vi "Examen01.vi"() -> ()   [LabVIEW 2020]
uses:
  <vilib>/Instr/_visa.llb/VISA Configure Serial Port (Instr).vi
panel:
  out "Waveform Chart":dynamicdata(graph)
  out "Valor Mínimo (°C)":dbl
  out "Valor Máximo (°C)":dbl
  out "Dato actual (°C)":dbl
  in  "stop":bool
  in  "VISA resource name":refnum<visa-resource-name>
  # "SENSOR LM35"
  # "Señal original"
  # "Señal filtrada"
  # "Juan Daniel Magdaleno Arellano\nLuis David Casas Hernandez"
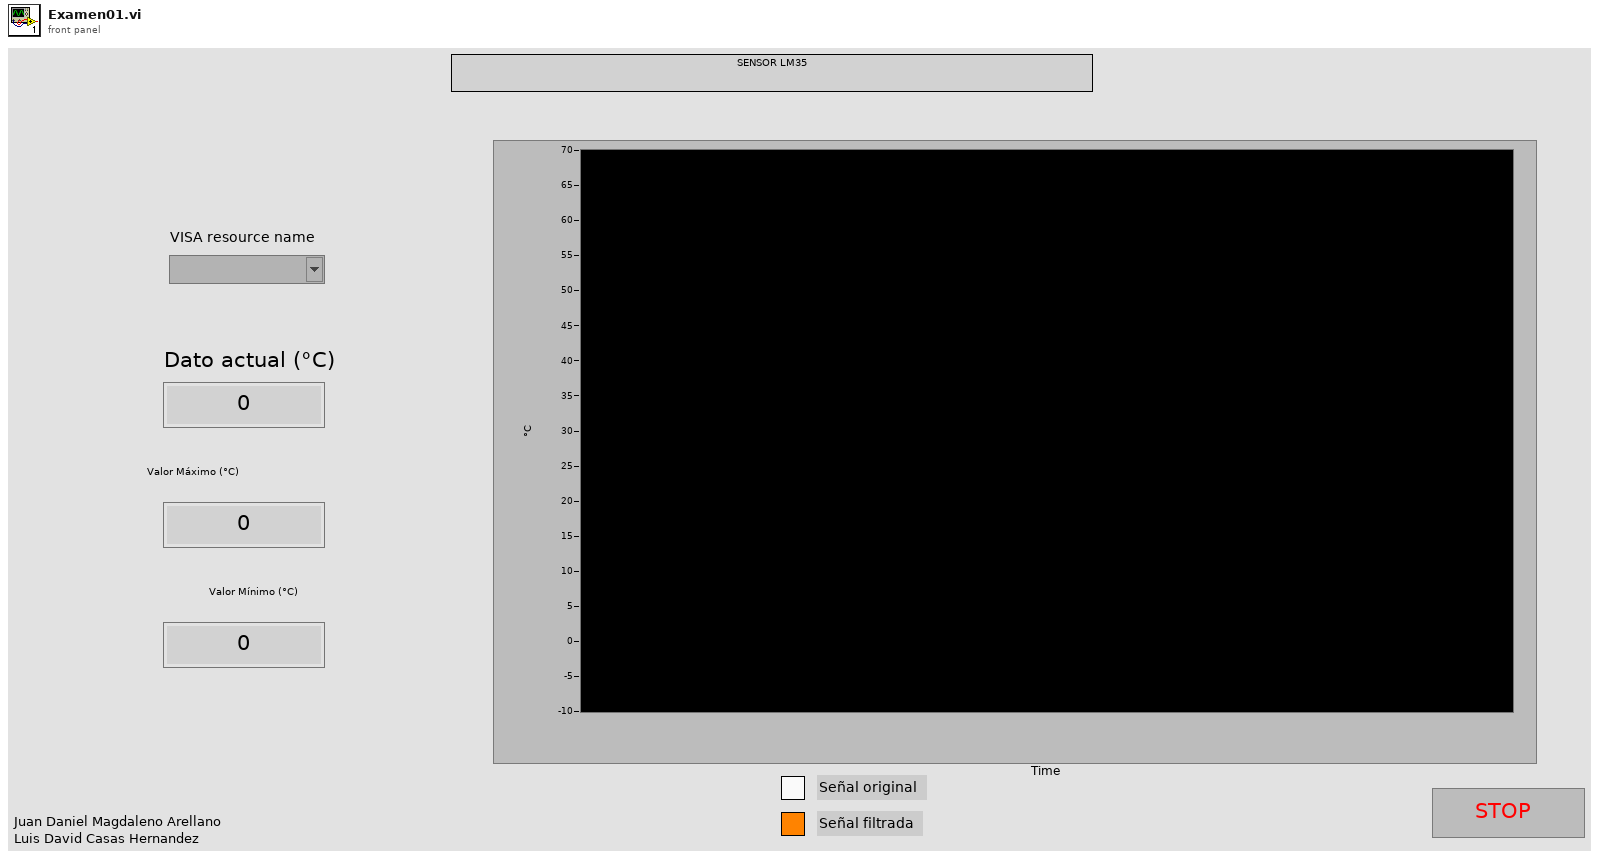
[diagram p1: front panel]
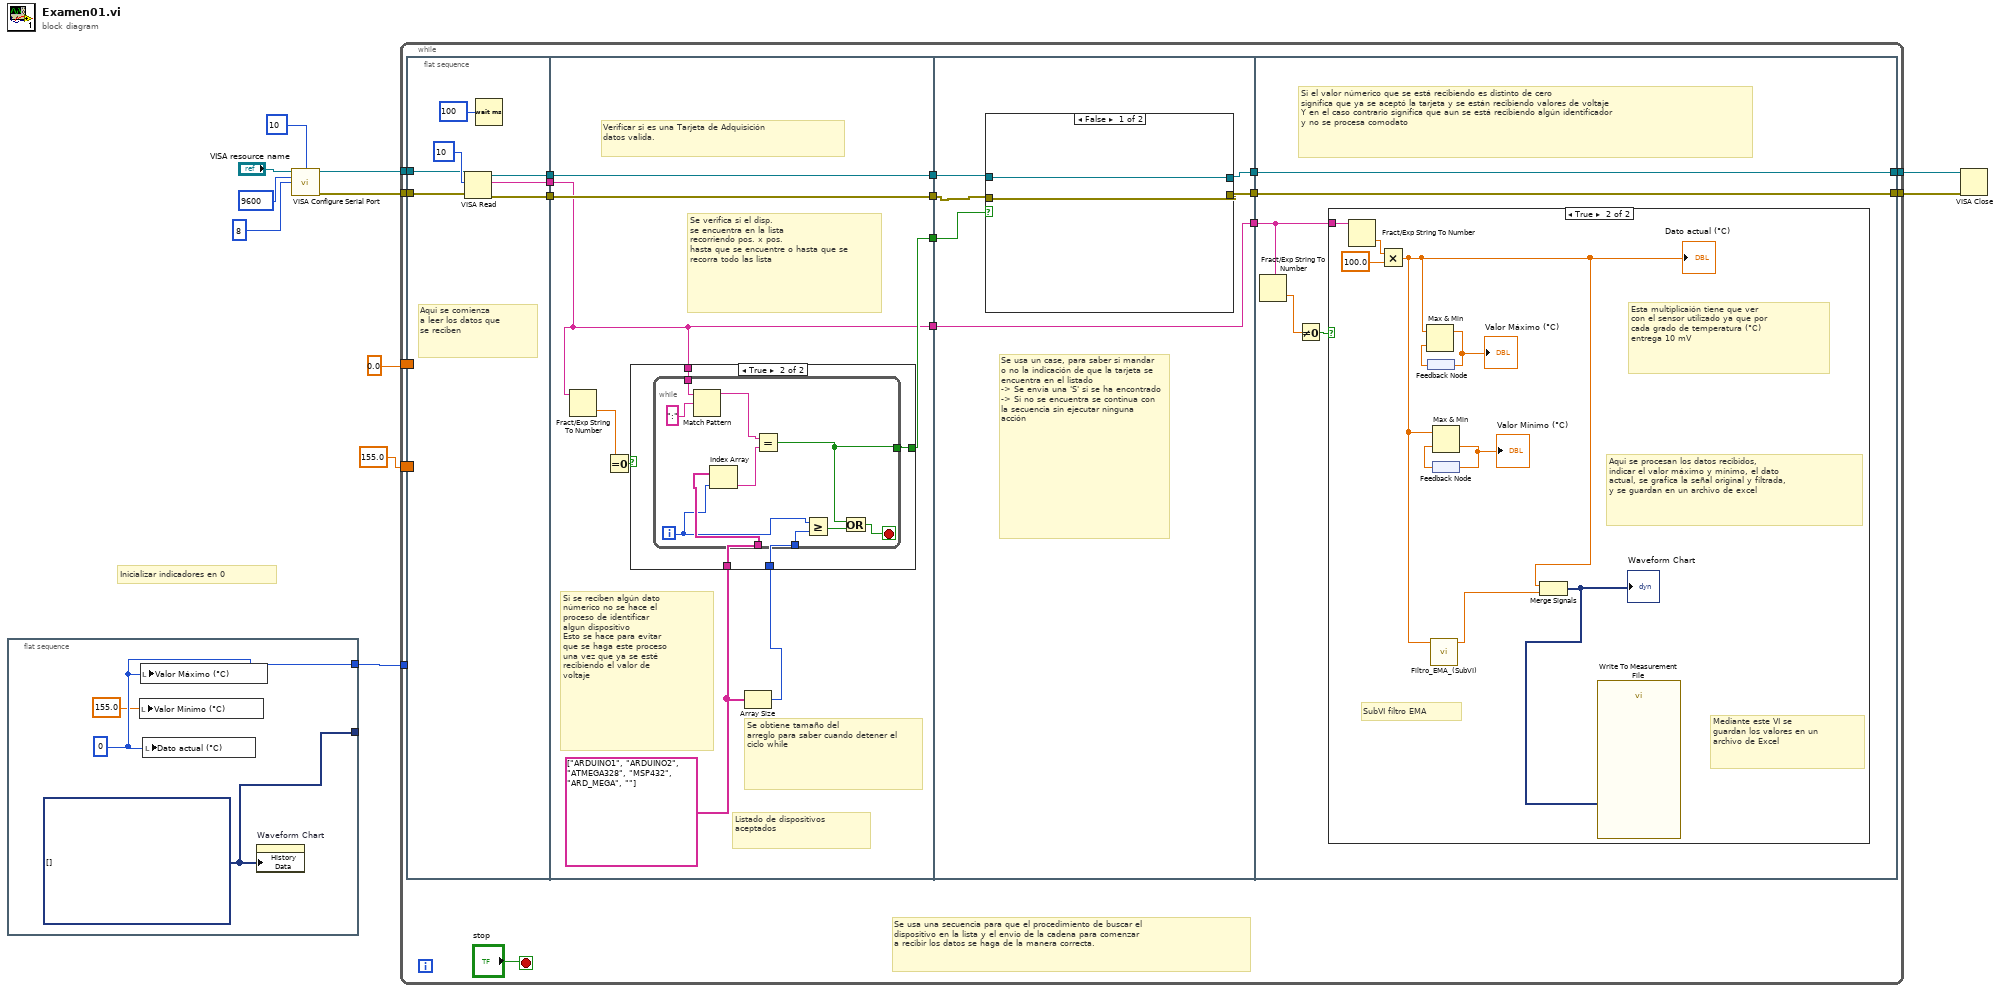
[diagram p0: block diagram]
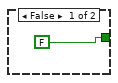
[diagram p2: hidden frame]
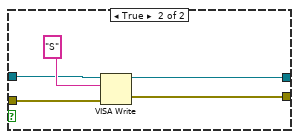
[diagram p3: hidden frame]
diagram:
  # "Inicializar indicadores en 0"
  n1 = flat-sequence {
    tunnel: [w14] -> w3
    tunnel: [w13] -> _
    frame #0 {
      w14 = 0
      w13 = dynamicdata[] [] ("History Data")
      n2 = local write "Valor Mínimo (°C)"(155.0) -> ()
      n3 = local write "Valor Máximo (°C)"(w14) -> ()
      n4 = local write "Dato actual (°C)"(w14) -> ()
      n5 = property on="Waveform Chart" class="WFChart (strict)"("History Data"=w13) -> ()  [unwired: 2 in, 2 out]
    }
  }
  n6 = call-poly "VISA Configure Serial Port"("VISA resource name"="VISA resource name", "termination char\n(0xA = '\\n' = LF)"=u8 10 ("termination char\n(0xA = '\\n' = LF)"), "baud rate (9600)"=u32 9600, "data bits (8)"=u16 8) -> ("VISA resource name out"=w11:refnum<visa-resource-name>, "error out"=w6:errorcluster)  [unwired: 10 in]
  n7 = while {
    tunnel: w11 -> [w20]
    tunnel: w6 -> [w19]
    tunnel: [w22] -> w5
    tunnel: [w21] -> w4
    tunnel: w3 -> [_]
    border: 0.0 -> [_]
    border: 155.0 -> [_]
    stop <- "stop" stop-if-true
    # "Se usa una secuencia para que el procedimiento de buscar el\ndispositivo en la lista y el envio de la cadena para comenzar\na recibir los datos se haga de la manera correcta."
    n8 = flat-sequence {
      tunnel: [w31] -> w28
      tunnel: [w32] -> w27
      tunnel: [w30] -> w26
      tunnel: w20 -> [w34]
      tunnel: w19 -> [w33]
      tunnel: w28 -> [w44]
      tunnel: w27 -> [w43]
      tunnel: w26 -> [w39]
      tunnel: [w44] -> w25
      tunnel: [w43] -> w24
      tunnel: [w40] -> w23
      tunnel: [w39] -> w18
      tunnel: w25 -> [w64]
      tunnel: w24 -> [w65]
      tunnel: w23 -> [w63]
      tunnel: [w62] -> w17
      tunnel: [w61] -> w16
      tunnel: [w60] -> w15
      tunnel: w18 -> [w60]
      tunnel: [w76] -> w21
      tunnel: [w77] -> w22
      tunnel: w17 -> [w77]
      tunnel: w16 -> [w76]
      tunnel: w15 -> [w75]
      frame #0 {
        # "Aqui se comienza\na leer los datos que\nse reciben"
        n9 = VISA Read(VISA resource name=w34, byte count=u32 10, error in (no error)=w33) -> (VISA resource name out=w32:refnum<visa-resource-name>, read buffer=w30:string, error out=w31:errorcluster)  [unwired: 1 out]
        n10 = Wait (ms)(milliseconds to wait=u32 100) -> ()  [unwired: 1 out]
      }
      frame #1 {
        w42 = string[] ["ARDUINO1", "ARDUINO2", "ATMEGA328", "MSP432", "ARD_MEGA", ""]
        # "Si se reciben algún dato\nnúmerico no se hace el\nproceso de identificar \nalgun dispositivo\nEsto se hace para evitar\nque se haga este proceso\nuna vez que ya se esté \nrecibiendo el valor de\nvoltaje"
        # "Se obtiene tamaño del\narreglo para saber cuando detener el\nciclo while"
        # "Se verifica si el disp.\nse encuentra en la lista\nrecorriendo pos. x pos.\nhasta que se encuentre o hasta que se recorra todo las lista"
        # "Listado de dispositivos\naceptados"
        # "Verificar si es una Tarjeta de Adquisición \ndatos valida."
        n11 = Fract/Exp String To Number(string=w39) -> (number=w37:dbl)  [unwired: 3 in, 1 out]
        n12 = Equal To 0?(x=w37) -> (x = 0?=w38:bool)
        n13 = Array Size(array=w42) -> (size(s)=w41:i32)
        n14 = case shown="True" w38 {
          tunnel: w42 -> [_ w49]
          tunnel: w41 -> [_ w48]
          tunnel: [FALSE w47] -> w40
          tunnel: w39 -> [_ w46]
          frame False {
          }
          frame True {
            n15 = while {
              tunnel: w49 -> [w56]
              tunnel: w48 -> [w59]
              tunnel: [w53] -> w47
              tunnel: w46 -> [w50]
              i -> [w55]
              stop <- w54 stop-if-true
              n16 = Match Pattern(string=w50, regular expression=":") -> (before substring=w51:string)  [unwired: 1 in, 3 out]
              n17 = Index Array(array=w56, index=w55) -> (element=w57:string)
              n18 = Equal?(x=w51, y=w57) -> (x = y?=w53:bool)
              n19 = Greater Or Equal?(x=w55, y=w59) -> (x >= y?=w58:bool)
              n20 = Or(x=w53, y=w58) -> (x .or. y?=w54:bool)
            }
          }
        }
      }
      frame #2 {
        # "Se usa un case, para saber si mandar o no la indicación de que la tarjeta se encuentra en el listado \n-> Se envia una 'S' si se ha encontrado\n-> Si no se encuentra se continua con la secuencia sin ejecutar ninguna acción"
        n21 = case shown="False" w63 {
          tunnel: [w66 w69] -> w61
          tunnel: [w67 w72] -> w62
          tunnel: w65 -> [w67 w70]
          tunnel: w64 -> [w66 w68]
          frame False {
          }
          frame True {
            n22 = VISA Write(VISA resource name=w70, write buffer="S", error in (no error)=w68) -> (VISA resource name out=w72:refnum<visa-resource-name>, error out=w69:errorcluster)  [unwired: 1 out]
          }
        }
      }
      frame #3 {
        # "Si el valor númerico que se está recibiendo es distinto de cero\nsignifica que ya se aceptó la tarjeta y se están recibiendo valores de voltaje\nY en el caso contrario significa que aun se está recibiendo algún identificador\ny no se procesa comodato"
        n23 = Fract/Exp String To Number(string=w75) -> (number=w74:dbl)  [unwired: 3 in, 1 out]
        n24 = Not Equal To 0?(x=w74) -> (x != 0?=w73:bool)
        n25 = case shown="True" w73 {
          tunnel: w75 -> [_ w87]
          frame False {
          }
          frame True {
            # "Mediante este VI se\nguardan los valores en un\narchivo de Excel"
            # "Esta multiplicaión tiene que ver\ncon el sensor utilizado ya que por\ncada grado de temperatura (°C)\nentrega 10 mV"
            # "SubVI filtro EMA"
            # "Aqui se procesan los datos recibidos,\nindicar el valor máximo y mínimo, el dato\nactual, se grafica la señal original y filtrada,\ny se guardan en un archivo de excel"
            n26 = Fract/Exp String To Number(string=w87) -> (number=w86:dbl)  [unwired: 3 in, 1 out]
            n27 = Multiply(x=w86, y=100.0) -> (x*y=w82:dbl)
            "Dato actual (°C)" <- w82
            n28 = feedback #1() -> (w83:dbl)
            n29 = Max & Min(x=w82, y=w83) -> (max(x,y)=w84:dbl)  [unwired: 1 out]
            "Valor Máximo (°C)" <- w84
            n30 = feedback-in #1(w84) -> ()
            n31 = call "Filtro_EMA_(SubVI).vi"("Entrada"=w82) -> ("Salida"=w81:dbl)  [unwired: 10 in]
            n32 = feedback #2() -> (w79:dbl)
            n33 = Max & Min(x=w82, y=w79) -> (min(x,y)=w78:dbl)  [unwired: 1 out]
            "Valor Mínimo (°C)" <- w78
            n34 = feedback-in #2(w78) -> ()
            n35 = Merge Signals "Merge Signals"(w82, w81) -> (w80:dynamicdata)
            "Waveform Chart" <- w80
            n36 = call "Write To Measurement File"("Signals"=w80) -> ()  [unwired: 16 in, 3 out]
          }
        }
      }
    }
  }
  n37 = VISA Close(VISA resource name=w5, error in (no error)=w4) -> ()  [unwired: 1 out]
